vi "4-10 easyRecorder.vi"() -> ()   [LabVIEW 2014]
doc: "------------------------------------\nAuther: Koji Ohashi\nCopyright (c) 2020 Japan LabVIEW Users Group, Volunteer members.\nThis VI is released under the MIT License.\nhttp://opensource.org/licenses/mit-license.php\n------------------------------------"
uses:
  4-10 ctl_easyRecorder/my_state.ctl
  <vilib>/sound2/lvsound2.llb/Sampling Mode.ctl
  <vilib>/sound2/lvsound2.llb/Sound Input Read (DBL).vi
  <vilib>/sound2/lvsound2.llb/Sound Output Write (DBL).vi
  <vilib>/sound2/lvsound2.llb/Sound Data Format.ctl
  <vilib>/Waveform/WDTOps.llb/WDT Number of Waveform Samples DBL.vi
panel:
  out "Filename Out":path
  in  "Radio Buttons":enum32{"Mic Input", "PC Sound"}(radio)
  in  "Process Stop Button":bool
  in  "Save As Button":bool
  in  "Open Button":bool
  in  "Play Button":bool
  in  "Record Button":bool
  out "Sound Input":waveform(dbl)[](graph)
  in  "Recording Time (sec)":dbl=5.0
  out "Number of Samples/ch":i32=10000
  out "my_state":T1
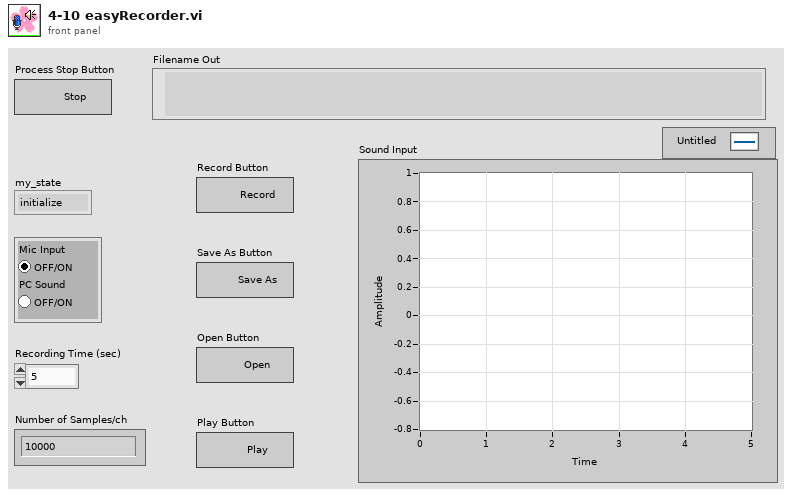
[diagram p1: front panel]
types:
  T1 = typedef "my_state.ctl" = enum16{"initialize", "stand by", "recording", "play", "save", "load", "end"}
  T2 = typedef "Sound Data Format.ctl" = cluster{"sample rate (S/s)":dbl, "number of channels":i32, "bits per sample":i32}
  T3 = typedef "Sampling Mode.ctl" = i32
  T4 = typedef "Sound Input Task ID.ctl" = u32
  T5 = typedef "Sound Output Task ID.ctl" = u32
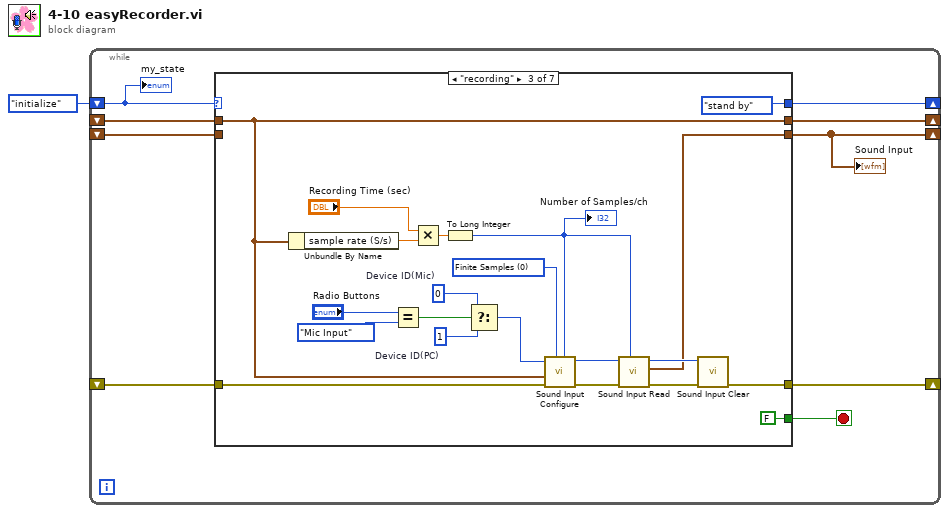
[diagram p0: block diagram]
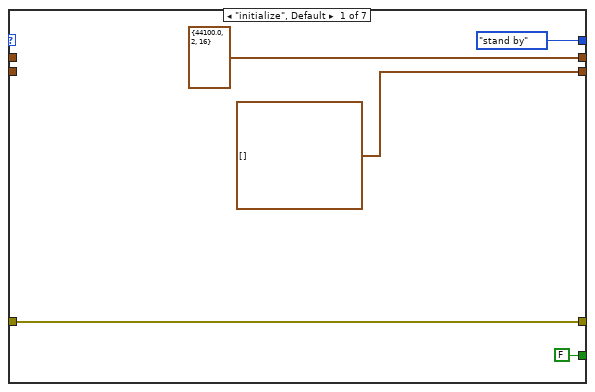
[diagram p2: hidden frame]
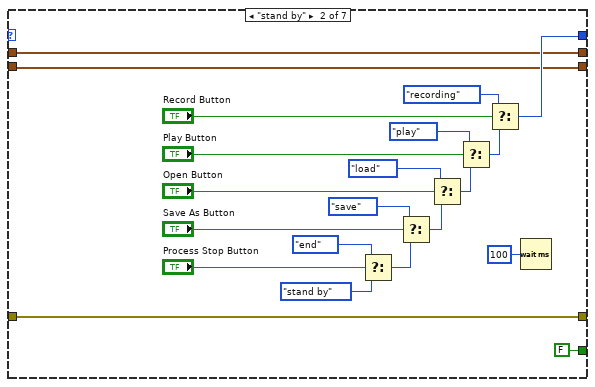
[diagram p3: hidden frame]
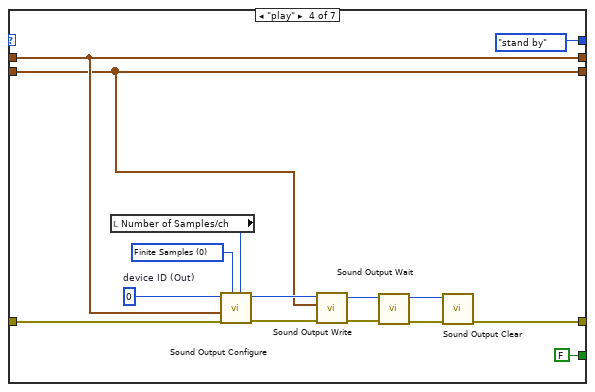
[diagram p4: hidden frame]
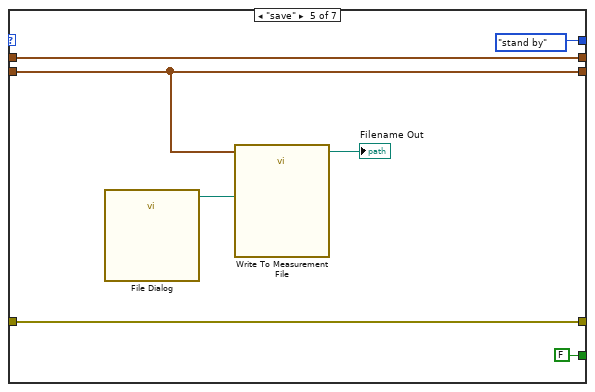
[diagram p5: hidden frame]
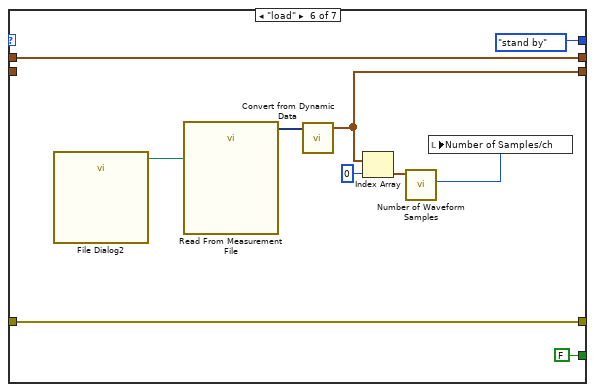
[diagram p6: hidden frame]
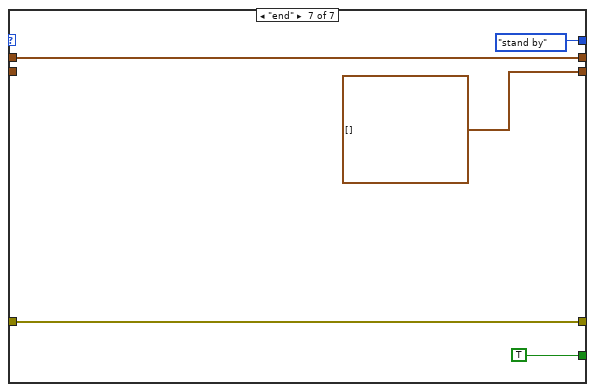
[diagram p7: hidden frame]
diagram:
  n1 = while {
    shift-right: [w10] -> _
    shift-left: my_state."initialize" ("my_state") -> [w6]
    shift-right: [w9] -> _
    shift-left: _ -> [w8]
    shift-right: [w2] -> _
    shift-left: _ -> [w5]
    shift-right: [w4] -> _
    shift-left: _ -> [w3]
    stop <- w7 stop-if-true
    n2 = case shown="\"recording\"" w6 {
      tunnel: [my_state."stand by" ("my_state") w26 my_state."stand by" ("my_state") my_state."stand by" ("my_state") my_state."stand by" ("my_state") my_state."stand by" ("my_state") my_state."stand by" ("my_state")] -> w10
      tunnel: [w14 w19 w46 w63 w78 w88 w92] -> w9
      tunnel: w8 -> [w14 w19 w47 w62 w78 w88 w92]
      tunnel: [FALSE FALSE FALSE FALSE FALSE FALSE TRUE] -> w7
      tunnel: [waveform(dbl)[] [] ("data") w16 w44 w59 w75 w81 waveform(dbl)[] [] ("data")] -> w2
      tunnel: w5 -> [_ w16 _ w59 w75 _ _]
      tunnel: [T2 {"sample rate (S/s)"=44100.0, "number of channels"=2, "bits per sample"=16} ("Sound Format") w17 w43 w60 w76 w86 w91] -> w4
      tunnel: w3 -> [_ w17 w43 w60 w76 w86 w91]
      frame "initialize", Default {
      }
      frame "stand by" {
        n3 = Select(t=my_state."end" ("my_state"), s="Process Stop Button", f=my_state."stand by" ("my_state")) -> (s? t:f=w22:T1)
        n4 = Select(t=my_state."save" ("my_state"), s="Save As Button", f=w22) -> (s? t:f=w21:T1)
        n5 = Select(t=my_state."load" ("my_state"), s="Open Button", f=w21) -> (s? t:f=w28:T1)
        n6 = Select(t=my_state."play" ("my_state"), s="Play Button", f=w28) -> (s? t:f=w27:T1)
        n7 = Select(t=my_state."recording" ("my_state"), s="Record Button", f=w27) -> (s? t:f=w26:T1)
        n8 = Wait (ms)(milliseconds to wait=u32 100) -> ()  [unwired: 1 out]
      }
      frame "recording" {
        w37 = u32 1  # Device ID(PC)
        w38 = u32 0  # Device ID(Mic)
        w54 = T3 0 items=["Finite Samples", "Continuous Samples"] ("sample mode")
        n9 = Unbundle By Name(w43) -> ("sample rate (S/s)"=w50:dbl)
        n10 = Equal?(x="Radio Buttons", y=enum32{"Mic Input", "PC Sound"}."Mic Input" ("Radio Buttons")) -> (x = y?=w39:bool)
        n11 = Multiply(x="Recording Time (sec)", y=w50) -> (x*y=w49:dbl)
        n12 = To Long Integer(number=w49) -> (32bit integer=w48:i32)
        "Number of Samples/ch" <- w48
        n13 = Select(t=w38, s=w39, f=w37) -> (s? t:f=w42:u32)
        n14 = call <vilib>:"Sound Input Configure.vi"("number of samples/ch"=w48, "sample mode"=w54, "error in (no error)"=w47, "sound format"=w43, "device ID"=w42) -> ("error out"=w56:errorcluster, "task ID"=w55:T4)  [unwired: 5 in]
        n15 = call-poly <vilib>:"Sound Input Read.vi"("number of samples/ch"=w48, "error in (no error)"=w56, "task ID"=w55) -> ("error out"=w52:errorcluster, "data"=w44:waveform(dbl)[], "task ID out"=w53:T4)  [unwired: 6 in]
        n16 = call <vilib>:"Sound Input Clear.vi"("error in (no error)"=w52, "task ID"=w53) -> ("error out"=w46:errorcluster)  [unwired: 9 in]
      }
      frame "play" {
        w71 = u32 0  # device ID (Out)
        w68 = T3 0 items=["Finite Samples", "Continuous Samples"] ("sample mode")
        n17 = local read "Number of Samples/ch"() -> (w58:i32)
        n18 = call <vilib>:"Sound Output Configure.vi"("number of samples/ch"=w58, "sample mode"=w68, "error in (no error)"=w62, "sound format"=w60, "device ID"=w71) -> ("error out"=w69:errorcluster, "task ID"=w70:T5)  [unwired: 5 in]
        n19 = call-poly <vilib>:"Sound Output Write.vi"("error in (no error)"=w69, "data"=w59, "task ID"=w70) -> ("error out"=w67:errorcluster, "task ID out"=w66:T5)  [unwired: 7 in]
        n20 = call <vilib>:"Sound Output Wait.vi"("error in (no error)"=w67, "task ID"=w66) -> ("error out"=w64:errorcluster, "task ID out"=w65:T5)  [unwired: 8 in]
        n21 = call <vilib>:"Sound Output Clear.vi"("error in (no error)"=w64, "task ID"=w65) -> ("error out"=w63:errorcluster)  [unwired: 9 in]
      }
      frame "save" {
        n22 = call "File Dialog"() -> ("selected path"=w73:path)  [unwired: 12 in, 3 out]
        n23 = call "Write To Measurement File"("Signals"=w75, "Filename"=w73) -> ("Filename Out"=→"Filename Out":path)  [unwired: 15 in, 2 out]
      }
      frame "load" {
        n24 = call "File Dialog2"() -> ("selected path"=w84:path)  [unwired: 12 in, 3 out]
        n25 = call "Read From Measurement File"("Filename"=w84) -> ("Signals"=w85:dynamicdata)  [unwired: 5 in, 5 out]
        n26 = call "Convert from Dynamic Data"("Dynamic Data Type"=w85) -> ("Array of Waveform"=w81:waveform(dbl)[])  [unwired: 3 in]
        n27 = Index Array(array=w81, index=0) -> (element=w82:waveform(dbl))
        n28 = call-poly <vilib>:"Number of Waveform Samples.vi"("waveform in"=w82) -> ("number of samples"=w80:i32)  [unwired: 8 in, 2 out]
        n29 = local write "Number of Samples/ch"(w80) -> ()
      }
      frame "end" {
      }
    }
    "Sound Input" <- w2
    "my_state" <- w6
  }
